vi "Demo HAL Tester LITE Auto.vi"() -> ()   [LabVIEW 2014]
doc: "Use this template to build a producer/consumer design pattern with events to produce queue items. Use this design pattern instead of the User Interface Event Handler pattern for user interfaces when you want to execute code asynchronously in response to an event without slowing the user interface responsiveness."
uses:
  TypeDefs/HAL Config Data.ctl
  APIs/Message Queue/Enqueue Message (Single).vi
  APIs/Message Queue/Enqueue Message (Array).vi
  APIs/Message Queue/WINFAS 2 Message Queue.lvlib
  HWSyncLoop/HWSyncLoop.lvlib
  APIs/Data Queue/WINFAS 2 Data Queue.lvlib
  HWAsyncLoop/HWAsyncLoop.lvlib
panel:
  out "Asyncs":string[][](array[string])
  out "Syncs":string[](array[string])
  out "Async Data":sgl[](array[numeric])
  in  "HWAsync CMD":bool
  in  "HWSync CMD":bool
  in  "Stop Cycle":bool
  in  "Start Cycle":bool
  in  "Config":bool
  in  "LOAD DRIVER":bool
  in  "Disconnect":bool
  in  "Connect":bool
  out "UI Mssge Log":string
  out "TDX":sgl[][](graph)
  out "Encoder":sgl[](array[slide]) scale=-3600.0..3600.0
  out "DO":bool[][](array[boolean])
  out "DI":bool[][](array[boolean])
  out "TDX ALL":string[][](table)
  out "HWSyncLog 1":string
  out "HWSyncLog 2":string
  out "HWSyncLog 3":string
  out "HWSyncLog 4":string
  out "HWSyncLog 5":string
  out "HWAsyncLogAll":string
  # "Entradas Digitales (0-15)"
  # "Salidas Digitales (0-15)"
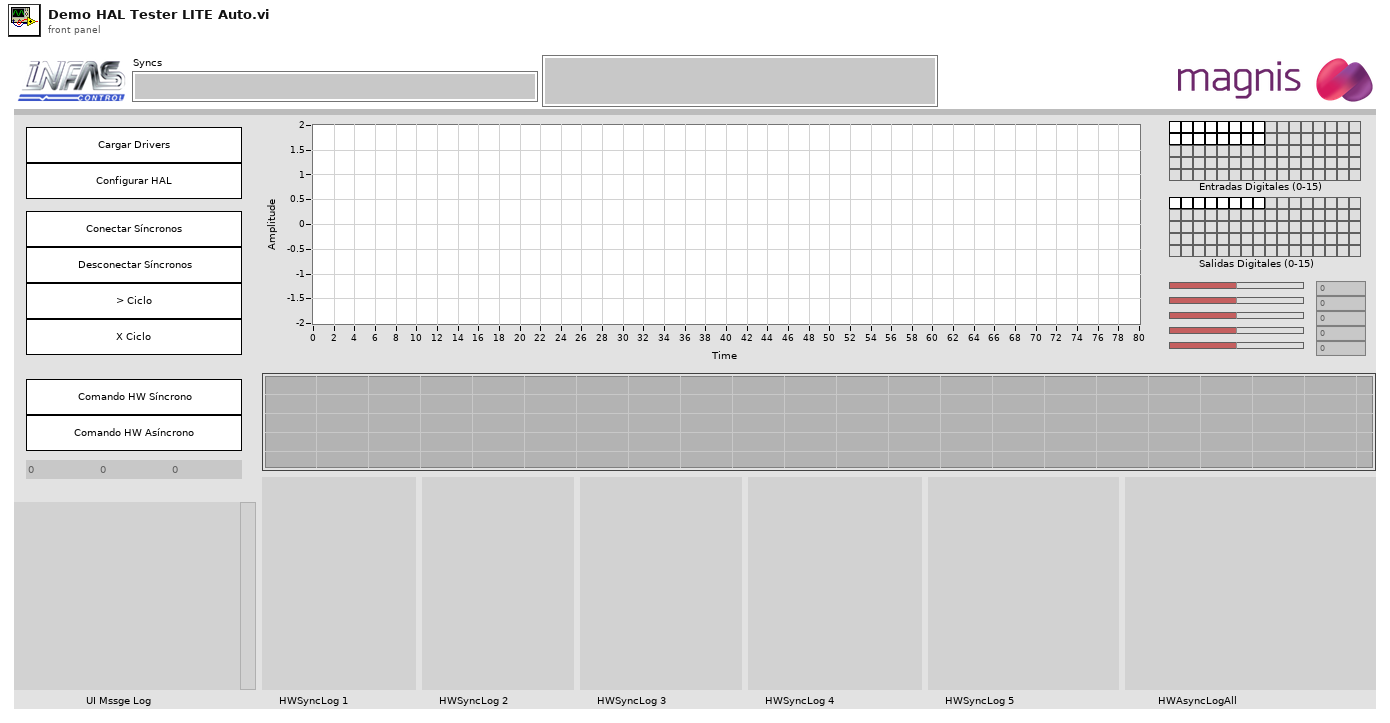
[diagram p1: front panel]
types:
  T1 = typedef "HAL Config Data.ctl" = cluster{"HWSync Index":u32, "Driver Name":string, "Channel Mask":u64}
  T2 = enum32{"invalid app kind", "Development System", "Run Time System", "Student Edition", "Embedded LabVIEW", "Evaluation", "Custom"}
  T3 = typedef "WINFAS 2 Message Queue.lvlib/All Message Queues.ctl" = cluster{"CORE":refnum<queue>, "Event UI":refnum<queue>, "Display UI":refnum<queue>, "MATH":refnum<queue>, "SEQ":refnum<queue>, "DB":refnum<queue>, "ERR":refnum<queue>, "HAL":refnum<queue>, "HWSync1":refnum<queue>, "HWSync2":refnum<queue>, "HWSync3":refnum<queue>, "HWSync4":refnum<queue>, "HWSync5":refnum<queue>, "HWAsync1":refnum<queue>, "HWAsync2":refnum<queue>, "HWAsync3":refnum<queue>, "HWAsync4":refnum<queue>, "HWAsync5":refnum<queue>, "HWAsync6":refnum<queue>, "HWAsync7":refnum<queue>, "HWAsync8":refnum<queue>, "HWAsync9":refnum<queue>, "HWAsync10":refnum<queue>}
  T4 = typedef "WINFAS 2 Data Queue.lvlib/All Data Queues Cluster.ctl" = cluster{"Queues":cluster{"ACQ HWSync1":refnum<queue>, "ACQ HWSync2":refnum<queue>, "ACQ HWSync3":refnum<queue>, "ACQ HWSync4":refnum<queue>, "ACQ HWSync5":refnum<queue>}, "Notifiers":cluster{"Control":cluster{"CTRL HWSync1":refnum<notifier>, "CTRL HWSync2":refnum<notifier>, "CTRL HWSync3":refnum<notifier>, "CTRL HWSync4":refnum<notifier>, "CTRL HWSync5":refnum<notifier>}, "Acquisition":cluster{"ACQ HWSync1":refnum<notifier>, "ACQ HWSync2":refnum<notifier>, "ACQ HWSync3":refnum<notifier>, "ACQ HWSync4":refnum<notifier>, "ACQ HWSync5":refnum<notifier>}, "Async":cluster{"ACQ HWAsync1":refnum<notifier>, "ACQ HWAsync2":refnum<notifier>, "ACQ HWAsync3":refnum<notifier>, "ACQ HWAsync4":refnum<notifier>, "ACQ HWAsync5":refnum<notifier>, "ACQ HWAsync6":refnum<notifier>, "ACQ HWAsync7":refnum<notifier>, "ACQ HWAsync8":refnum<notifier>, "ACQ HWAsync9":refnum<notifier>, "ACQ HWAsync10":refnum<notifier>}}}
  T5 = cluster{"ACQ HWSync1":refnum<notifier>, "ACQ HWSync2":refnum<notifier>, "ACQ HWSync3":refnum<notifier>, "ACQ HWSync4":refnum<notifier>, "ACQ HWSync5":refnum<notifier>}
  T6 = cluster{"CTRL HWSync1":refnum<notifier>, "CTRL HWSync2":refnum<notifier>, "CTRL HWSync3":refnum<notifier>, "CTRL HWSync4":refnum<notifier>, "CTRL HWSync5":refnum<notifier>}
  T7 = cluster{"ACQ HWSync1":refnum<queue>, "ACQ HWSync2":refnum<queue>, "ACQ HWSync3":refnum<queue>, "ACQ HWSync4":refnum<queue>, "ACQ HWSync5":refnum<queue>}
  T8 = cluster{"HWSync1":refnum<queue>, "HWSync2":refnum<queue>, "HWSync3":refnum<queue>, "HWSync4":refnum<queue>, "HWSync5":refnum<queue>}
  T9 = cluster{"HWAsync1":refnum<queue>, "HWAsync2":refnum<queue>, "HWAsync3":refnum<queue>, "HWAsync4":refnum<queue>, "HWAsync5":refnum<queue>, "HWAsync6":refnum<queue>, "HWAsync7":refnum<queue>, "HWAsync8":refnum<queue>, "HWAsync9":refnum<queue>, "HWAsync10":refnum<queue>}
  T10 = typedef "WINFAS 2 Data Queue.lvlib/Async Acquisition Data Cluster.ctl" = cluster{"Data":sgl[]}
  T11 = typedef "WINFAS 2 Data Queue.lvlib/Acquisition Data 1 Sample Cluster.ctl" = cluster{"TDX":sgl[], "Encoder":sgl}
  T12 = typedef "WINFAS 2 Data Queue.lvlib/Control Data Cluster.ctl" = cluster{"Encoder":sgl, "DI":bool[], "DO":bool[]}
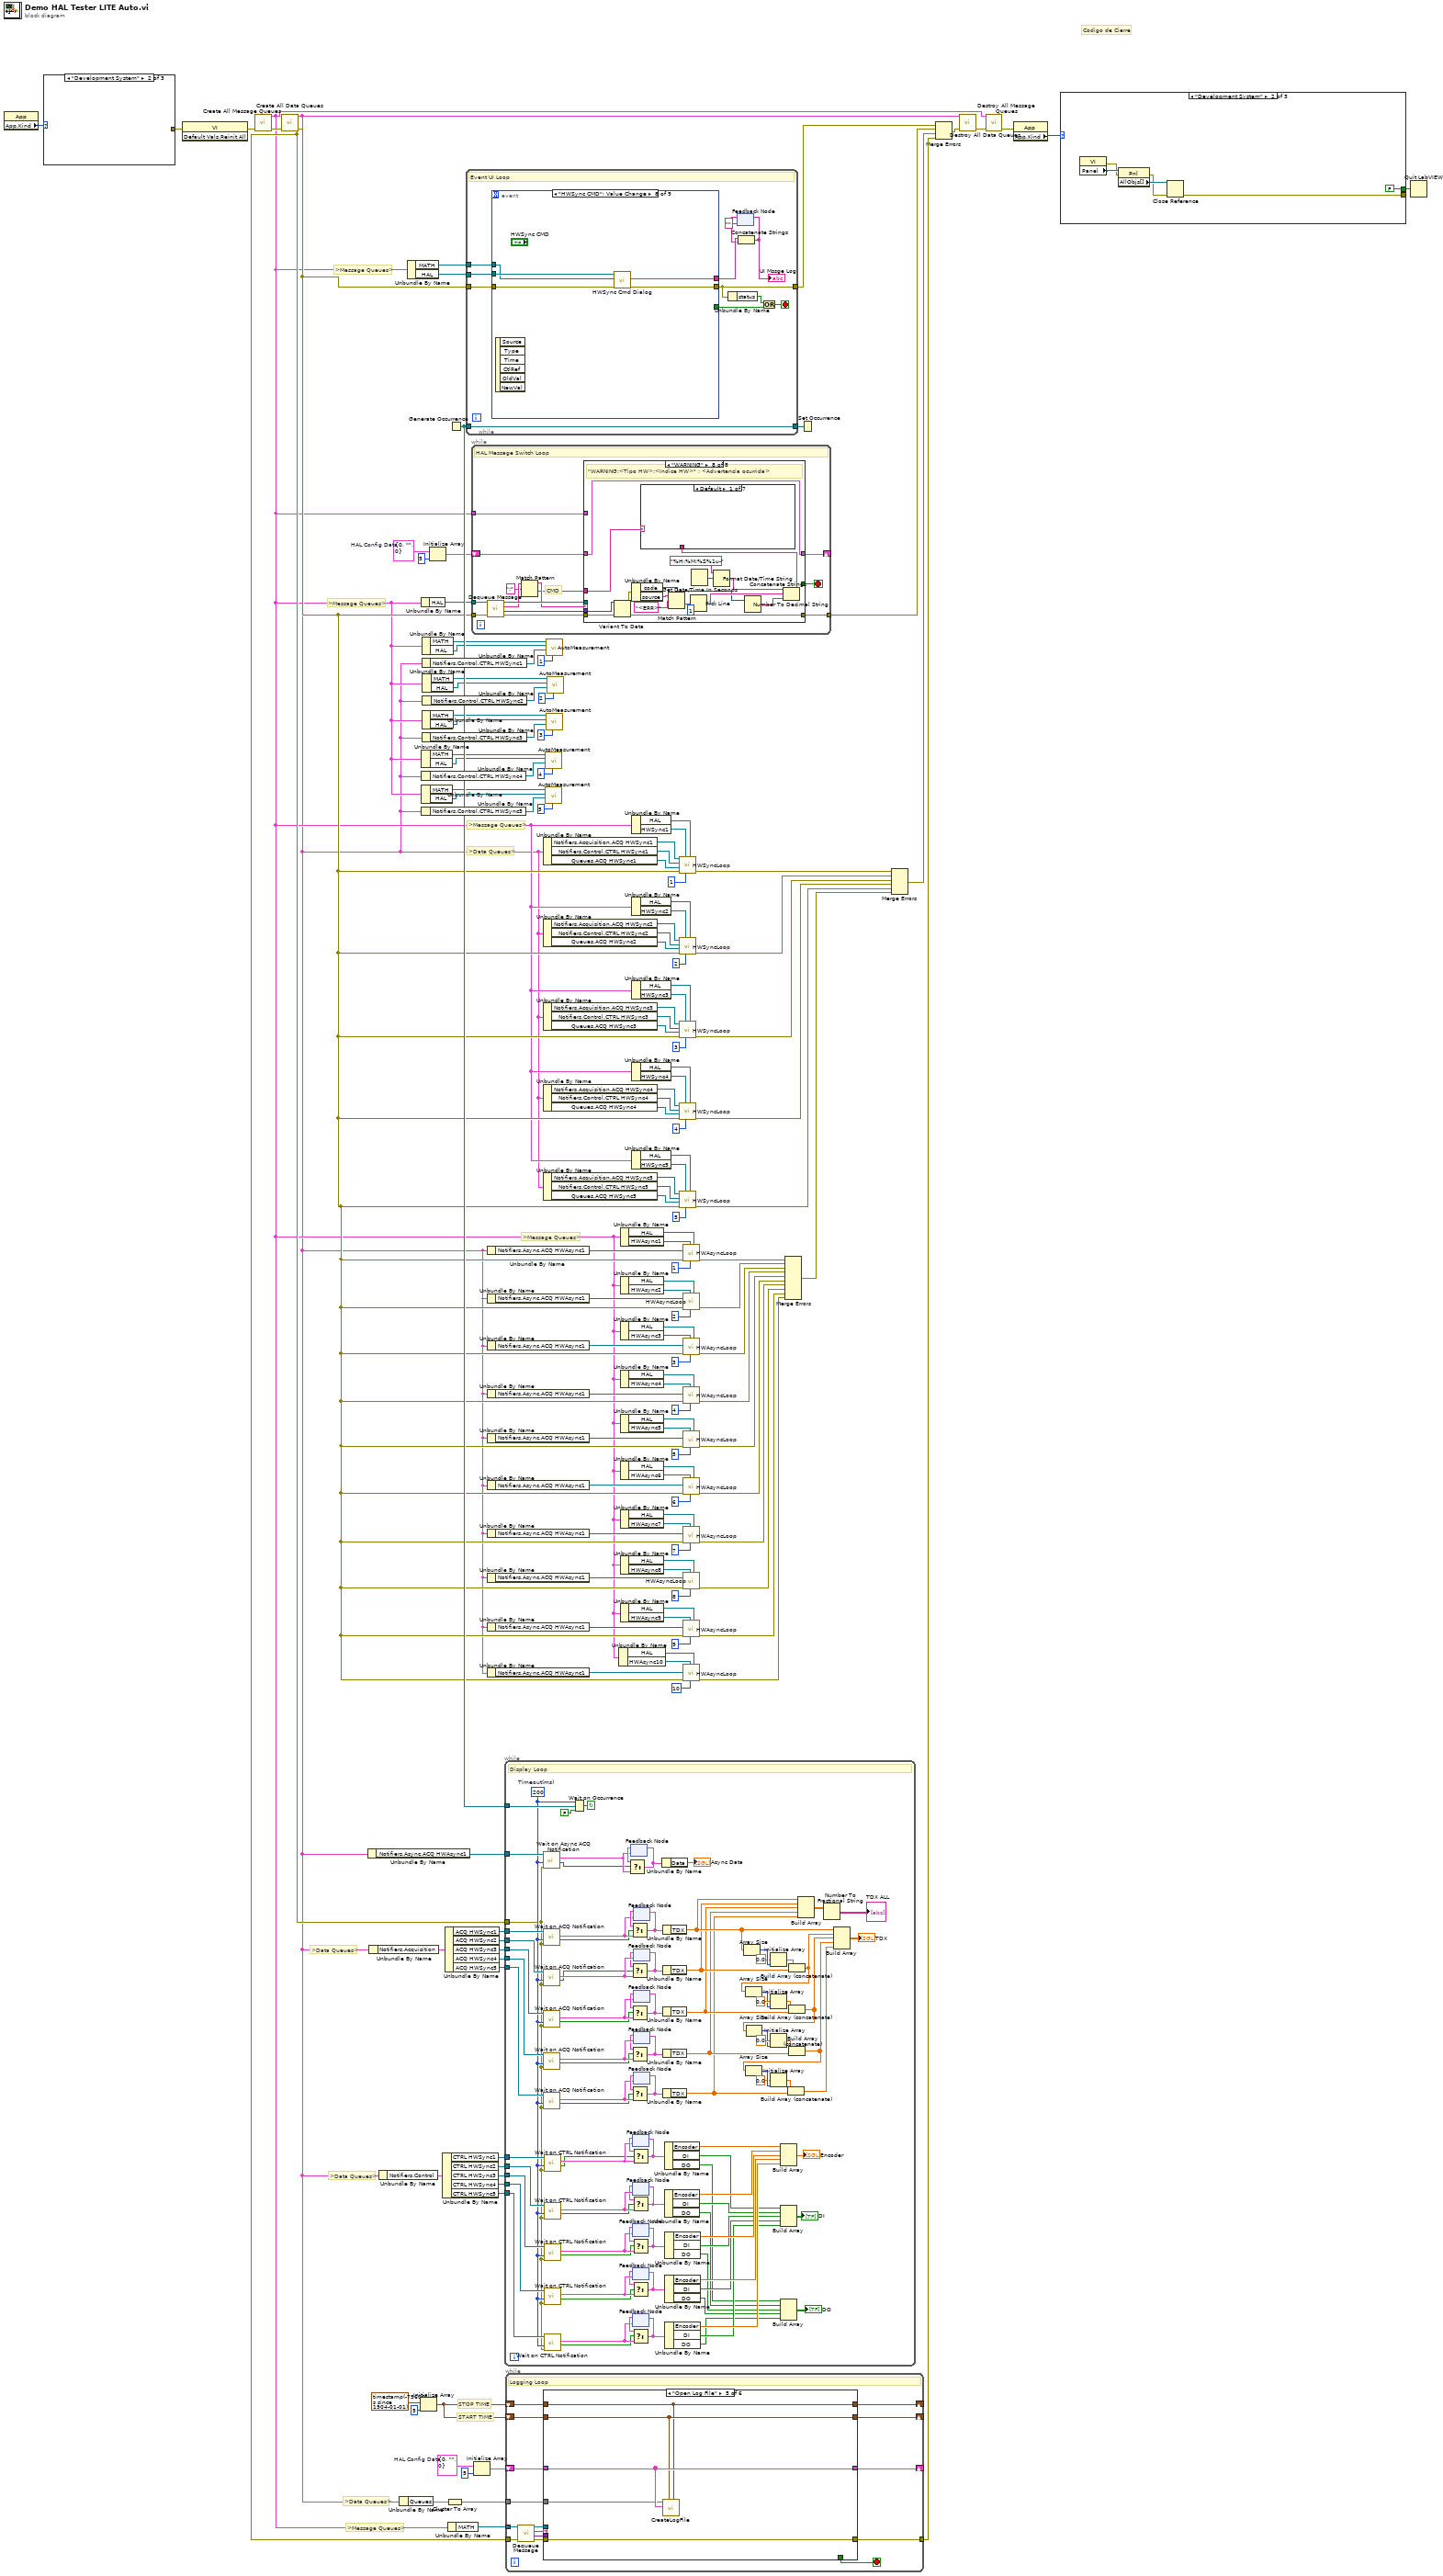
[diagram p0: block diagram]
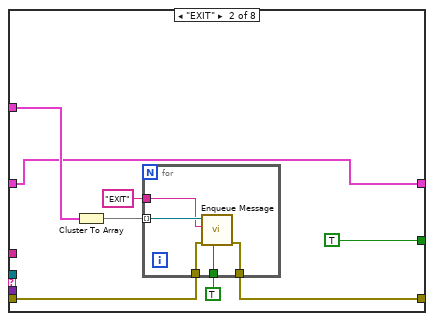
[diagram p3: hidden frame]
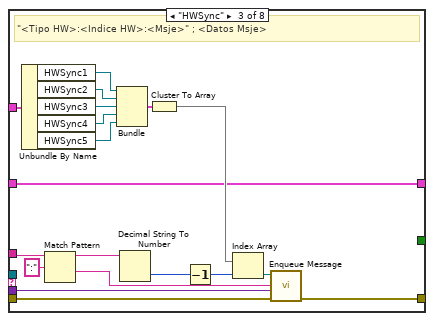
[diagram p4: hidden frame]
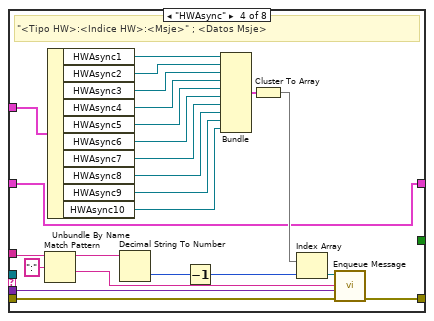
[diagram p5: hidden frame]
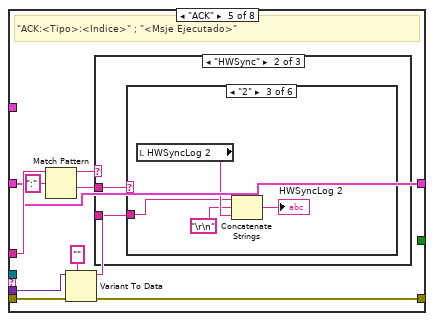
[diagram p6: hidden frame]
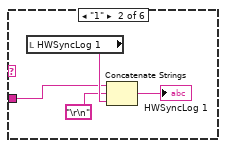
[diagram p9: hidden frame]
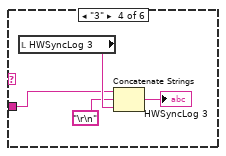
[diagram p10: hidden frame]
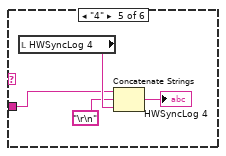
[diagram p11: hidden frame]
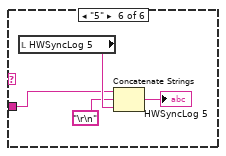
[diagram p12: hidden frame]
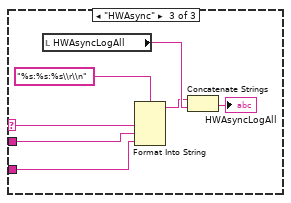
[diagram p13: hidden frame]
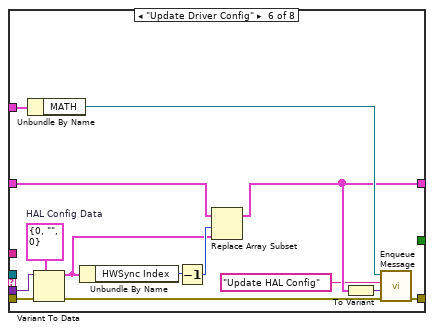
[diagram p14: hidden frame]
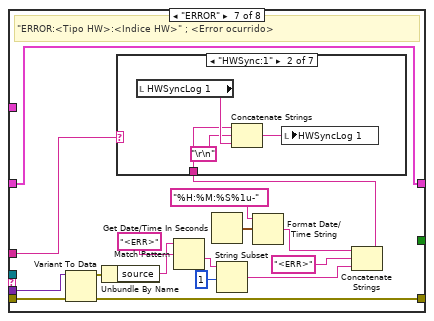
[diagram p15: hidden frame]
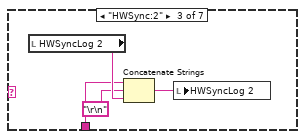
[diagram p17: hidden frame]
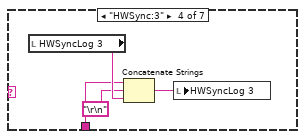
[diagram p18: hidden frame]
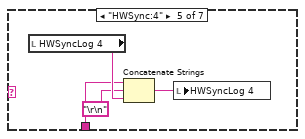
[diagram p19: hidden frame]
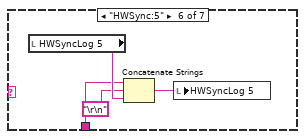
[diagram p20: hidden frame]
diagram:
  w39 = T1 {"HWSync Index"=0, "Driver Name"="", "Channel Mask"=0}  # HAL Config Data
  w42 = T1 {"HWSync Index"=0, "Driver Name"="", "Channel Mask"=0}  # HAL Config Data
  # "START TIME"
  # "STOP TIME"
  # ">Message Queues>"
  # ">Message Queues>"
  # ">Data Queues>"
  # "Codigo de Cierre"
  # ">Message Queues>"
  # ">Data Queues>"
  # ">Message Queues>"
  # ">Data Queues>"
  # ">Data Queues>"
  # ">Message Queues>"
  n1 = property class="App"() -> ("App.Kind"=w143:T2)  [unwired: 2 in, 2 out]
  n2 = case shown="\"Development System\"" w143 {
    tunnel: [_ _ w154] -> w142
    frame "invalid app kind", Default {
    }
    frame "Development System" {
    }
    frame "Run Time System" {
      w153 = FALSE ("Front Panel Window:Show Menu Bar")
      n3 = invoke class="VI" method="FP.Run-Time Position.Maximized"("Monitor"=i16 0) -> (error out=w154:errorcluster)  [unwired: 3 in, 3 out]
      n4 = property class="VI"("Front Panel.ShowMenuBar"=w153, "TB.Visible"=w153) -> ()  [unwired: 2 in, 2 out]
    }
  }
  n5 = invoke class="VI" method="Default Vals.Reinit All"(error in=w142) -> (error out=w133:errorcluster)  [unwired: 2 in, 2 out]
  n6 = call "Create All Message Queues.vi"("error in (no error)"=w133) -> ("error out"=w134:errorcluster, "Message Queues Out"=w2:T3)  [unwired: 9 in]
  n7 = call "Create All Data Queues.vi"("Error In"=w134) -> ("Error Out"=w57:errorcluster, "WINFAS 2 Data Queue.lvlib:All Data Queues Cluster"=w1:T4)  [unwired: 9 in]
  n8 = Unbundle By Name(w1) -> ("Notifiers.Async.ACQ HWAsync1"=w24:refnum<notifier>)
  n9 = Unbundle By Name(w1) -> ("Notifiers.Acquisition"=w89:T5)
  n10 = Unbundle By Name(w1) -> ("Notifiers.Control"=w88:T6)
  n11 = Unbundle By Name(w1) -> ("Queues"=w36:T7)
  n12 = Unbundle By Name(w2) -> ("MATH"=w152:refnum<queue>, "HAL"=w148:refnum<queue>)
  n13 = Initialize Array(timestamp(-75600 s since 1904-01-01) ("current time"), 5 ("dimension size")) -> (w43:timestamp[])
  n14 = Unbundle By Name(w2) -> ("HAL"=w23:refnum<queue>)
  n15 = Unbundle By Name(w2) -> ("MATH"=w7:refnum<queue>, "HAL"=w8:refnum<queue>)
  n16 = Unbundle By Name(w1) -> ("Notifiers.Control.CTRL HWSync4"=w9:refnum<notifier>)
  n17 = Unbundle By Name(w2) -> ("MATH"=w6:refnum<queue>, "HAL"=w5:refnum<queue>)
  n18 = Unbundle By Name(w1) -> ("Notifiers.Control.CTRL HWSync5"=w4:refnum<notifier>)
  n19 = Unbundle By Name(w2) -> ("MATH"=w22:refnum<queue>, "HAL"=w21:refnum<queue>)
  n20 = Unbundle By Name(w1) -> ("Notifiers.Control.CTRL HWSync1"=w20:refnum<notifier>)
  n21 = Unbundle By Name(w2) -> ("MATH"=w14:refnum<queue>, "HAL"=w13:refnum<queue>)
  n22 = Unbundle By Name(w1) -> ("Notifiers.Control.CTRL HWSync3"=w12:refnum<notifier>)
  n23 = Unbundle By Name(w2) -> ("MATH"=w15:refnum<queue>, "HAL"=w16:refnum<queue>)
  n24 = Unbundle By Name(w1) -> ("Notifiers.Control.CTRL HWSync2"=w17:refnum<notifier>)
  n25 = Initialize Array(w39, 5 ("dimension size")) -> (w37:T1[])
  n26 = Unbundle By Name(w88) -> ("CTRL HWSync1"=w97:refnum<notifier>, "CTRL HWSync2"=w96:refnum<notifier>, "CTRL HWSync3"=w95:refnum<notifier>, "CTRL HWSync4"=w94:refnum<notifier>, "CTRL HWSync5"=w93:refnum<notifier>)
  n27 = Unbundle By Name(w89) -> ("ACQ HWSync1"=w138:refnum<notifier>, "ACQ HWSync2"=w101:refnum<notifier>, "ACQ HWSync3"=w100:refnum<notifier>, "ACQ HWSync4"=w99:refnum<notifier>, "ACQ HWSync5"=w98:refnum<notifier>)
  n28 = Cluster To Array(cluster=w36) -> (array=w35:refnum<queue>[])
  n29 = Unbundle By Name(w2) -> ("MATH"=w146:refnum<queue>)
  n30 = Generate Occurrence() -> (w131:refnum<k4>)
  n31 = while {
    tunnel: w152 -> [w167]
    tunnel: w148 -> [w162]
    tunnel: [w160] -> w132
    tunnel: w131 -> [w160]
    tunnel: w57 -> [w166]
    tunnel: [w164] -> w149
    stop <- w161 stop-if-true
    # "Event UI Loop"
    n32 = event shown="[7] \"HWSync CMD\": Value Change" {
      selector: _ -> [_ _ _ _ _ _ _ _ _]
      dyn-events: _ -> [_ _ _ _ _ _ _ _ _]
      timeout: _ -> [_ _ _ _ _ _ _ _ _]
      tunnel: w167 -> [w173 _ _ _ _ _ w232 w247 _]
      tunnel: w166 -> [w175 w185 w191 w200 w207 w214 w231 w251 w257]
      tunnel: [w170 w183 w190 w199 w206 w212 w236 w250 w255] -> w164
      tunnel: [TRUE ("stop") _ _ _ _ _ _ _ _] -> w165
      tunnel: w162 -> [w176 w184 w189 w198 w205 w213 w237 w249 w252]
      tunnel: [_ w182 w186 w195 w204 w209 w235 w248 w254] -> w159
      event Panel Close? {
        w174 = TRUE ("Priority Message? (F)")
        w172 = "EXIT" ("String")
        n33 = event-data() -> ()  [unwired: 1 in, 1 out]
        n34 = call-poly "Enqueue Message.vi"("Priority Message? (F)"=w174, "error in (no error)"=w175, "Message"=w172, "Message Queue"=w176) -> ("error out"=w171:errorcluster)  [unwired: 6 in, 1 out]
        n35 = call-poly "Enqueue Message.vi"("Priority Message? (F)"=w174, "error in (no error)"=w171, "Message"=w172, "Message Queue"=w173) -> ("error out"=w170:errorcluster)  [unwired: 6 in, 1 out]
        n36 = event-data("Discard?"=TRUE) -> ()  [unwired: 1 in, 1 out]
      }
      event "LOAD DRIVER": Value Change {
        n37 = event-data() -> ()  [unwired: 1 in, 1 out]
        n38 = call "Load Drivers Dialog.vi"("error in (no error)"=w185, "Message Queue in"=w184) -> ("error out"=w183:errorcluster, "Mssgs Sent"=w182:string, "Asyncs"=w180:string[], "Syncs"=→"Syncs":string[])  [unwired: 6 in]
        n39 = Reshape Array(w180, 2 ("dimension size"), 5 ("dimension size")) -> (→"Asyncs":string[][])
      }
      event "Connect": Value Change {
        w188 = string[] ["HWSync:1:Port:Open", "HWSync:2:Port:Open", "HWSync:3:Port:Open", "HWSync:4:Port:Open", "HWSync:5:Port:Open"] ("Message Array")
        n40 = event-data() -> ()  [unwired: 1 in, 1 out]
        n41 = for {
          tunnel: [w194] -> w187 mode=indexing
          tunnel: w188 -> [w193] mode=indexing
          n42 = Concatenate Strings(w193, "\r\n") -> (w194:string)
        }
        n43 = call-poly "Enqueue Message.vi"("error in (no error)"=w191, "Message Array"=w188, "Message Queue"=w189) -> ("error out"=w190:errorcluster)  [unwired: 7 in, 1 out]
        n44 = Concatenate Strings(w187) -> (w186:string)
      }
      event "Disconnect": Value Change {
        w196 = string[] ["HWSync:1:Port:Close", "HWSync:2:Port:Close", "HWSync:3:Port:Close", "HWSync:4:Port:Close", "HWSync:5:Port:Close"] ("Message Array")
        n45 = event-data() -> ()  [unwired: 1 in, 1 out]
        n46 = for {
          tunnel: [w203] -> w197 mode=indexing
          tunnel: w196 -> [w202] mode=indexing
          n47 = Concatenate Strings(w202, "\r\n") -> (w203:string)
        }
        n48 = call-poly "Enqueue Message.vi"("error in (no error)"=w200, "Message Array"=w196, "Message Queue"=w198) -> ("error out"=w199:errorcluster)  [unwired: 7 in, 1 out]
        n49 = Concatenate Strings(w197) -> (w195:string)
      }
      event "Config": Value Change {
        n50 = event-data() -> ()  [unwired: 1 in, 1 out]
        n51 = call "Config Select Dialog.vi"("Error In"=w207, "Message Queue"=w205) -> ("Error Out"=w206:errorcluster, "Msg out"=w204:string)  [unwired: 8 in]
      }
      event "Start Cycle": Value Change {
        n52 = event-data() -> ()  [unwired: 1 in, 2 out]
        n53 = for {
          N: 5 -> [_]
          tunnel: w213 -> [w228]
          shift-right: [w227] -> w212
          shift-left: w214 -> [w229]
          tunnel: [w218] -> w210 mode=concatenating
          i -> [w226]
          n54 = Increment(x=w226) -> (x+1=w222:i32)
          n55 = Format Into String(format string="HWSync:%d:Auto-Refresh:Init" ("String"), w222) -> (resulting string=w221:string)  [unwired: 2 in, 1 out]
          n56 = Format Into String(format string="HWSync:%d:Auto-Refresh:Start" ("String"), w222) -> (resulting string=w220:string)  [unwired: 2 in, 1 out]
          n57 = Format Into String(format string="HWSync:%d:Diagnostic:Cycle" ("String"), w222) -> (resulting string=w219:string)  [unwired: 2 in, 1 out]
          n58 = Build Array(w221, w220, w219) -> (w218:string[])
          n59 = call-poly "Enqueue Message.vi"("error in (no error)"=w229, "Message Array"=w218, "Message Queue"=w228) -> ("error out"=w227:errorcluster)  [unwired: 7 in, 1 out]
        }
        n60 = for {
          tunnel: [w217] -> w211 mode=indexing
          tunnel: w210 -> [w216] mode=indexing
          n61 = Concatenate Strings(w216, "\r\n") -> (w217:string)
        }
        n62 = Concatenate Strings(w211) -> (w209:string)
      }
      event "Stop Cycle": Value Change {
        n63 = event-data() -> ()  [unwired: 1 in, 1 out]
        n64 = for {
          N: 5 -> [_]
          tunnel: w237 -> [w245]
          shift-right: [w244] -> w236
          shift-left: w231 -> [w246]
          tunnel: [w238] -> w234 mode=indexing
          i -> [w243]
          n65 = Increment(x=w243) -> (x+1=w241:i32)
          n66 = Format Into String(format string="HWSync:%d:Auto-Refresh:Stop" ("String"), w241) -> (resulting string=w239:string)  [unwired: 2 in, 1 out]
          n67 = call-poly "Enqueue Message.vi"("error in (no error)"=w246, "Message"=w239, "Message Queue"=w245) -> ("error out"=w244:errorcluster)  [unwired: 7 in, 1 out]
          n68 = Concatenate Strings(w239, "\r\n") -> (w238:string)
        }
        n69 = call-poly "Enqueue Message.vi"("error in (no error)"=w231, "Message"="Open Log File", "Message Queue"=w232) -> ()  [unwired: 7 in, 2 out]
        n70 = Concatenate Strings(w234) -> (w235:string)
      }
      event "HWSync CMD": Value Change {
        n71 = event-data() -> ()  [unwired: 1 in, 6 out]
        n72 = call "HWSync Cmd Dialog.vi"("error in (no error)"=w251, "Log Queue"=w247, "Hal Queue in"=w249) -> ("error out"=w250:errorcluster, "Msg out"=w248:string)  [unwired: 7 in]
      }
      event "HWAsync CMD": Value Change {
        n73 = event-data() -> ()  [unwired: 1 in, 6 out]
        n74 = call "HWAsync Cmd Dialog.vi"("error in (no error)"=w257) -> ("error out"=w256:errorcluster, "Msg out"=w253:string)  [unwired: 9 in]
        n75 = call "HWAsync Cmd END Dialog.vi"("error in (no error)"=w256, "Msg in"=w253, "Message Queue"=w252) -> ("error out"=w255:errorcluster, "Msg out"=w254:string)  [unwired: 7 in]
      }
    }
    n76 = Unbundle By Name(w164) -> ("status"=w163:bool)
    n77 = feedback #1("") -> (w158:string)
    n78 = Concatenate Strings(w159, w158) -> (w157:string)
    "UI Mssge Log" <- w157
    n79 = feedback-in #1(w157) -> ()
    n80 = Or(x=w163, y=w165) -> (x .or. y?=w161:bool)
  }
  n81 = while {
    tunnel: w23 -> [w271]
    tunnel: w57 -> [w270]
    tunnel: [w262] -> w90
    tunnel: w2 -> [w261]
    shift-right: [w258] -> _
    shift-left: w37 -> [w259]
    stop <- w266 stop-if-true
    # "CMD"
    # "HAL Message Switch Loop"
    n82 = call "Dequeue Message.vi"("error in (no error)"=w270, "Message Queue"=w271) -> ("error out"=w269:errorcluster, "Message Data"=w268:variant, "Message"=w265:string, "dup Message Queue"=w267:refnum<queue>)  [unwired: 6 in]
    n83 = Match Pattern(string=w265, regular expression=":") -> (before substring=w263:string, after substring=w260:string)  [unwired: 1 in, 2 out]
    n84 = case shown="\"WARNING\"" w263 {
      tunnel: w269 -> [w273 w280 w305 w329 w339 w382 w389 w436]
      tunnel: w268 -> [_ _ w303 w327 w338 w381 w398 w441]
      tunnel: w267 -> [_ _ _ _ _ _ _ _]
      tunnel: [_ TRUE _ _ _ _ _ _] -> w266
      tunnel: [w273 w279 w304 w328 w337 w374 w397 w440] -> w262
      tunnel: w261 -> [_ w277 w302 w326 _ w373 _ _]
      tunnel: w260 -> [_ _ w295 w320 w333 _ w386 w434]
      tunnel: w259 -> [w272 w274 w287 w306 w330 w376 w385 w433]
      tunnel: [w272 w274 w287 w306 w330 w370 w385 w433] -> w258
      frame Default {
      }
      frame "EXIT" {
        n85 = Cluster To Array(cluster=w277) -> (array=w276:refnum<queue>[])
        n86 = for {
          tunnel: w276 -> [w284] mode=indexing
          tunnel: "EXIT" ("regular expression") -> [w283]
          tunnel: w280 -> [w286]
          tunnel: [w285] -> w279
          tunnel: TRUE -> [w282]
          n87 = call-poly "Enqueue Message.vi"("Priority Message? (F)"=w282, "error in (no error)"=w286, "Message"=w283, "Message Queue"=w284) -> ("error out"=w285:errorcluster)  [unwired: 6 in, 1 out]
        }
      }
      frame "HWSync" {
        # "\"<Tipo HW>:<Indice HW>:<Msje>\" ; <Datos Msje>"
        n88 = Unbundle By Name(w302) -> ("HWSync1"=w298:refnum<queue>, "HWSync2"=w300:refnum<queue>, "HWSync3"=w301:refnum<queue>, "HWSync4"=w299:refnum<queue>, "HWSync5"=w297:refnum<queue>)
        n89 = Match Pattern(string=w295, regular expression=":") -> (before substring=w292:string, after substring=w290:string)  [unwired: 1 in, 2 out]
        n90 = Bundle("HWSync1"=w298, "HWSync2"=w300, "HWSync3"=w301, "HWSync4"=w299, "HWSync5"=w297) -> (w294:T8)  [unwired: 1 in]
        n91 = Decimal String To Number(string=w292) -> (number=w288:i32)  [unwired: 2 in, 1 out]
        n92 = Cluster To Array(cluster=w294) -> (array=w293:refnum<queue>[])
        n93 = Decrement(x=w288) -> (x-1=w289:i32)
        n94 = Index Array(array=w293, index=w289) -> (element=w291:refnum<queue>)
        n95 = call-poly "Enqueue Message.vi"("error in (no error)"=w305, "Message Data"=w303, "Message"=w290, "Message Queue"=w291) -> ("error out"=w304:errorcluster)  [unwired: 6 in, 1 out]
      }
      frame "HWAsync" {
        # "\"<Tipo HW>:<Indice HW>:<Msje>\" ; <Datos Msje>"
        n96 = Match Pattern(string=w320, regular expression=":") -> (before substring=w317:string, after substring=w315:string)  [unwired: 1 in, 2 out]
        n97 = Unbundle By Name(w326) -> ("HWAsync1"=w323:refnum<queue>, "HWAsync2"=w307:refnum<queue>, "HWAsync3"=w325:refnum<queue>, "HWAsync4"=w324:refnum<queue>, "HWAsync5"=w322:refnum<queue>, "HWAsync6"=w308:refnum<queue>, "HWAsync7"=w309:refnum<queue>, "HWAsync8"=w310:refnum<queue>, "HWAsync9"=w311:refnum<queue>, "HWAsync10"=w312:refnum<queue>)
        n98 = Decimal String To Number(string=w317) -> (number=w313:i32)  [unwired: 2 in, 1 out]
        n99 = Decrement(x=w313) -> (x-1=w314:i32)
        n100 = Bundle("HWAsync1"=w323, "HWAsync2"=w307, "HWAsync3"=w325, "HWAsync4"=w324, "HWAsync5"=w322, "HWAsync6"=w308, "HWAsync7"=w309, "HWAsync8"=w310, "HWAsync9"=w311, "HWAsync10"=w312) -> (w319:T9)  [unwired: 1 in]
        n101 = Cluster To Array(cluster=w319) -> (array=w318:refnum<queue>[])
        n102 = Index Array(array=w318, index=w314) -> (element=w316:refnum<queue>)
        n103 = call-poly "Enqueue Message.vi"("error in (no error)"=w329, "Message Data"=w327, "Message"=w315, "Message Queue"=w316) -> ("error out"=w328:errorcluster)  [unwired: 6 in, 1 out]
      }
      frame "ACK" {
        # "\"ACK:<Tipo>:<Indice>\" ; \"<Msje Ejecutado>\""
        n104 = Match Pattern(string=w333, regular expression=":") -> (before substring=w334:string, after substring=w331:string)  [unwired: 1 in, 2 out]
        n105 = Variant To Data(error in=w339, type="", Variant=w338) -> (data=w336:string, error out=w337:errorcluster)
        n106 = case shown="\"HWSync\"" w334 {
          selector: w334 -> [_ _ w367]
          tunnel: w336 -> [_ w341 w365]
          tunnel: w331 -> [_ w340 w366]
          frame Default {
          }
          frame "HWSync" {
            n107 = case shown="\"2\"" w340 {
              tunnel: w341 -> [_ w342 w348 w352 w356 w360]
              frame Default {
              }
              frame "1" {
                n108 = local read "HWSyncLog 1"() -> (w345:string)
                n109 = Concatenate Strings(w342, "\r\n", w345) -> (→"HWSyncLog 1":string)
              }
              frame "2" {
                n110 = local read "HWSyncLog 2"() -> (w349:string)
                n111 = Concatenate Strings(w348, "\r\n", w349) -> (→"HWSyncLog 2":string)
              }
              frame "3" {
                n112 = local read "HWSyncLog 3"() -> (w353:string)
                n113 = Concatenate Strings(w352, "\r\n", w353) -> (→"HWSyncLog 3":string)
              }
              frame "4" {
                n114 = local read "HWSyncLog 4"() -> (w357:string)
                n115 = Concatenate Strings(w356, "\r\n", w357) -> (→"HWSyncLog 4":string)
              }
              frame "5" {
                n116 = local read "HWSyncLog 5"() -> (w361:string)
                n117 = Concatenate Strings(w360, "\r\n", w361) -> (→"HWSyncLog 5":string)
              }
            }
          }
          frame "HWAsync" {
            n118 = local read "HWAsyncLogAll"() -> (w364:string)
            n119 = Format Into String(format string="%s:%s:%s\\r\\n", w367, w366, w365) -> (resulting string=w363:string)  [unwired: 2 in, 1 out]
            n120 = Concatenate Strings(w363, w364) -> (→"HWAsyncLogAll":string)
          }
        }
      }
      frame "Update Driver Config" {
        w380 = T1 {"HWSync Index"=0, "Driver Name"="", "Channel Mask"=0}  # HAL Config Data
        n121 = Unbundle By Name(w373) -> ("MATH"=w372:refnum<queue>)
        n122 = Variant To Data(error in=w382, type=w380, Variant=w381) -> (data=w377:T1, error out=w375:errorcluster)
        n123 = Unbundle By Name(w377) -> ("HWSync Index"=w379:u32)
        n124 = Decrement(x=w379) -> (x-1=w378:u32)
        n125 = Replace Array Subset(array=w376, new element=w377, index=w378) -> (w370:T1[])
        n126 = To Variant(anything=w370) -> (Variant=w371:variant)
        n127 = call-poly "Enqueue Message.vi"("error in (no error)"=w375, "Message Data"=w371, "Message"="Update HAL Config" ("regular expression"), "Message Queue"=w372) -> ("error out"=w374:errorcluster)  [unwired: 6 in, 1 out]
      }
      frame "ERROR" {
        # "\"ERROR:<Tipo HW>:<Indice HW>\" ; <Error ocurrido>"
        n128 = Variant To Data(error in=w389, type=w389, Variant=w398) -> (data=w388:errorcluster, error out=w397:errorcluster)
        n129 = Unbundle By Name(w388) -> ("source"=w395:string)
        n130 = Match Pattern(string=w395, regular expression="<ERR>") -> (after substring=w391:string)  [unwired: 1 in, 3 out]
        n131 = Get Date/Time In Seconds() -> (seconds since 1Jan1904=w394:timestamp)
        n132 = String Subset(string=w391, offset (0)=1) -> (substring=w384:string)  [unwired: 1 in]
        n133 = Format Date/Time String(time format string (%c)="%H:%M:%S%1u-", seconds (now)=w394) -> (date/time string=w392:string)  [unwired: 1 in]
        n134 = Concatenate Strings(w392, "<ERR>" ("string"), w384) -> (w387:string)
        n135 = case shown="\"HWSync:1\"" w386 {
          selector: w386 -> [_ _ _ _ _ _ w422]
          tunnel: w387 -> [_ w401 w405 w409 w413 w417 w424]
          frame Default {
          }
          frame "HWSync:1" {
            n136 = local read "HWSyncLog 1"() -> (w402:string)
            n137 = Concatenate Strings(w401, "\r\n", w402) -> (w399:string)
            n138 = local write "HWSyncLog 1"(w399) -> ()
          }
          frame "HWSync:2" {
            n139 = local read "HWSyncLog 2"() -> (w406:string)
            n140 = Concatenate Strings(w405, "\r\n", w406) -> (w403:string)
            n141 = local write "HWSyncLog 2"(w403) -> ()
          }
          frame "HWSync:3" {
            n142 = local read "HWSyncLog 3"() -> (w410:string)
            n143 = Concatenate Strings(w409, "\r\n", w410) -> (w407:string)
            n144 = local write "HWSyncLog 3"(w407) -> ()
          }
          frame "HWSync:4" {
            n145 = local read "HWSyncLog 4"() -> (w414:string)
            n146 = Concatenate Strings(w413, "\r\n", w414) -> (w411:string)
            n147 = local write "HWSyncLog 4"(w411) -> ()
          }
          frame "HWSync:5" {
            n148 = local read "HWSyncLog 5"() -> (w418:string)
            n149 = Concatenate Strings(w417, "\r\n", w418) -> (w415:string)
            n150 = local write "HWSyncLog 5"(w415) -> ()
          }
          frame "HWAsync:1", "HWAsync:10", "HWAsync:2", "HWAsync:3", "HWAsync:4", "HWAsync:5", "HWAsync:6", "HWAsync:7", "HWAsync:8", "HWAsync:9" {
            n151 = local read "HWAsyncLogAll"() -> (w419:string)
            n152 = Concatenate Strings(w422, ":" ("string"), w424, "\r\n", w419) -> (w420:string)
            n153 = local write "HWAsyncLogAll"(w420) -> ()
          }
        }
      }
      frame "WARNING" {
        # "\"WARNING:<Tipo HW>:<Indice HW>\" ; <Advertencia ocurrida>"
        n154 = Variant To Data(error in=w436, type=w436, Variant=w441) -> (data=w431:errorcluster, error out=w440:errorcluster)
        n155 = Unbundle By Name(w431) -> ("code"=w426:i32, "source"=w430:string)
        n156 = Match Pattern(string=w430, regular expression="<ERR>") -> (after substring=w428:string)  [unwired: 1 in, 3 out]
        n157 = Pick Line(multi-line string=w428, line index=1) -> (output string=w427:string)  [unwired: 1 in]
        n158 = Get Date/Time In Seconds() -> (seconds since 1Jan1904=w439:timestamp)
        n159 = Format Date/Time String(time format string (%c)="%H:%M:%S%1u-", seconds (now)=w439) -> (date/time string=w437:string)  [unwired: 1 in]
        n160 = Number To Decimal String(number=w426) -> (decimal integer string=w432:string)  [unwired: 1 in]
        n161 = Concatenate Strings(w437, w427, w432) -> (w435:string)
        n162 = case shown="Default" w434 {
          selector: w434 -> [_ _ _ _ _ _ w465]
          tunnel: w435 -> [_ w444 w448 w452 w456 w460 w467]
          frame Default {
          }
          frame "HWSync:1" {
            n163 = local read "HWSyncLog 1"() -> (w445:string)
            n164 = Concatenate Strings(w444, "\r\n", w445) -> (w442:string)
            n165 = local write "HWSyncLog 1"(w442) -> ()
          }
          frame "HWSync:2" {
            n166 = local read "HWSyncLog 2"() -> (w449:string)
            n167 = Concatenate Strings(w448, "\r\n", w449) -> (w446:string)
            n168 = local write "HWSyncLog 2"(w446) -> ()
          }
          frame "HWSync:3" {
            n169 = local read "HWSyncLog 3"() -> (w453:string)
            n170 = Concatenate Strings(w452, "\r\n", w453) -> (w450:string)
            n171 = local write "HWSyncLog 3"(w450) -> ()
          }
          frame "HWSync:4" {
            n172 = local read "HWSyncLog 4"() -> (w457:string)
            n173 = Concatenate Strings(w456, "\r\n", w457) -> (w454:string)
            n174 = local write "HWSyncLog 4"(w454) -> ()
          }
          frame "HWSync:5" {
            n175 = local read "HWSyncLog 5"() -> (w461:string)
            n176 = Concatenate Strings(w460, "\r\n", w461) -> (w458:string)
            n177 = local write "HWSyncLog 5"(w458) -> ()
          }
          frame "HWAsync:1", "HWAsync:10", "HWAsync:2", "HWAsync:3", "HWAsync:4", "HWAsync:5", "HWAsync:6", "HWAsync:7", "HWAsync:8", "HWAsync:9" {
            n178 = local read "HWAsyncLogAll"() -> (w462:string)
            n179 = Concatenate Strings(w465, ":" ("string"), w467, "\r\n", w462) -> (w463:string)
            n180 = local write "HWAsyncLogAll"(w463) -> ()
          }
        }
      }
    }
  }
  n181 = Initialize Array(w42, 5 ("dimension size")) -> (w40:T1[])
  n182 = Unbundle By Name(w1) -> ("Notifiers.Async.ACQ HWAsync1"=w34:refnum<notifier>)
  n183 = Unbundle By Name(w1) -> ("Notifiers.Async.ACQ HWAsync1"=w33:refnum<notifier>)
  n184 = Unbundle By Name(w1) -> ("Notifiers.Async.ACQ HWAsync1"=w32:refnum<notifier>)
  n185 = Unbundle By Name(w1) -> ("Notifiers.Async.ACQ HWAsync1"=w31:refnum<notifier>)
  n186 = Unbundle By Name(w1) -> ("Notifiers.Async.ACQ HWAsync1"=w30:refnum<notifier>)
  n187 = Unbundle By Name(w1) -> ("Notifiers.Async.ACQ HWAsync1"=w29:refnum<notifier>)
  n188 = Unbundle By Name(w1) -> ("Notifiers.Async.ACQ HWAsync1"=w28:refnum<notifier>)
  n189 = Unbundle By Name(w1) -> ("Notifiers.Async.ACQ HWAsync1"=w27:refnum<notifier>)
  n190 = Unbundle By Name(w1) -> ("Notifiers.Async.ACQ HWAsync1"=w26:refnum<notifier>)
  n191 = Unbundle By Name(w1) -> ("Notifiers.Async.ACQ HWAsync1"=w25:refnum<notifier>)
  n192 = while {
    tunnel: w138 -> [w570]
    tunnel: w131 -> [w564]
    tunnel: w101 -> [w549]
    tunnel: w100 -> [w548]
    tunnel: w99 -> [w547]
    tunnel: w98 -> [w546]
    tunnel: w57 -> [w483]
    tunnel: w97 -> [w515]
    tunnel: w96 -> [w514]
    tunnel: w95 -> [w513]
    tunnel: w94 -> [w512]
    tunnel: w93 -> [w511]
    tunnel: w24 -> [w485]
    stop <- w565 continue-if-true
    w484 = 200  # Timeout(ms)
    # "Display Loop"
    n193 = call "Wait on Async ACQ Notification.vi"("error in (no error)"=w483, "timeout in ms (-1)"=w484, "Async ACQ Notifier in"=w485) -> ("timed out?"=w478:bool, "Async ACQ"=w481:T10)  [unwired: 5 in, 2 out]
    n194 = call "Wait on ACQ Notification.vi"("error in (no error)"=w483, "timeout in ms (-1)"=w484, "ACQ Data Notifier in"=w570) -> ("timed out?"=w477:bool, "1 Sample"=w563:T11)  [unwired: 5 in, 2 out]
    n195 = call "Wait on ACQ Notification.vi"("error in (no error)"=w483, "timeout in ms (-1)"=w484, "ACQ Data Notifier in"=w549) -> ("timed out?"=w476:bool, "1 Sample"=w561:T11)  [unwired: 5 in, 2 out]
    n196 = call "Wait on ACQ Notification.vi"("error in (no error)"=w483, "timeout in ms (-1)"=w484, "ACQ Data Notifier in"=w548) -> ("timed out?"=w475:bool, "1 Sample"=w556:T11)  [unwired: 5 in, 2 out]
    n197 = call "Wait on ACQ Notification.vi"("error in (no error)"=w483, "timeout in ms (-1)"=w484, "ACQ Data Notifier in"=w547) -> ("timed out?"=w474:bool, "1 Sample"=w555:T11)  [unwired: 5 in, 2 out]
    n198 = call "Wait on ACQ Notification.vi"("error in (no error)"=w483, "timeout in ms (-1)"=w484, "ACQ Data Notifier in"=w546) -> ("timed out?"=w473:bool, "1 Sample"=w550:T11)  [unwired: 5 in, 2 out]
    n199 = call "Wait on CTRL Notification.vi"("error in (no error)"=w483, "timeout in ms (-1)"=w484, "CTRL Data Notifier in"=w515) -> ("timed out?"=w472:bool, "Control Data"=w562:T12)  [unwired: 5 in, 2 out]
    n200 = call "Wait on CTRL Notification.vi"("error in (no error)"=w483, "timeout in ms (-1)"=w484, "CTRL Data Notifier in"=w514) -> ("timed out?"=w471:bool, "Control Data"=w543:T12)  [unwired: 5 in, 2 out]
    n201 = call "Wait on CTRL Notification.vi"("error in (no error)"=w483, "timeout in ms (-1)"=w484, "CTRL Data Notifier in"=w513) -> ("timed out?"=w470:bool, "Control Data"=w538:T12)  [unwired: 5 in, 2 out]
    n202 = call "Wait on CTRL Notification.vi"("error in (no error)"=w483, "timeout in ms (-1)"=w484, "CTRL Data Notifier in"=w512) -> ("timed out?"=w469:bool, "Control Data"=w537:T12)  [unwired: 5 in, 2 out]
    n203 = call "Wait on CTRL Notification.vi"("error in (no error)"=w483, "timeout in ms (-1)"=w484, "CTRL Data Notifier in"=w511) -> ("timed out?"=w468:bool, "Control Data"=w532:T12)  [unwired: 5 in, 2 out]
    n204 = Wait on Occurrence(1:FALSE ("ignore previous (T)"), 2:w564, 3:w484) -> (0:w565:bool)
    n205 = feedback #2(w481) -> (w482:T10)
    n206 = Select(t=w482, s=w478, f=w481) -> (s? t:f=w480:T10)
    n207 = feedback-in #2(w480) -> ()
    n208 = feedback #3(w562) -> (w569:T12)
    n209 = Select(t=w569, s=w472, f=w562) -> (s? t:f=w568:T12)
    n210 = feedback-in #3(w568) -> ()
    n211 = feedback #4(w543) -> (w541:T12)
    n212 = Select(t=w541, s=w471, f=w543) -> (s? t:f=w542:T12)
    n213 = feedback-in #4(w542) -> ()
    n214 = feedback #5(w538) -> (w540:T12)
    n215 = Select(t=w540, s=w470, f=w538) -> (s? t:f=w539:T12)
    n216 = feedback-in #5(w539) -> ()
    n217 = feedback #6(w537) -> (w535:T12)
    n218 = Select(t=w535, s=w469, f=w537) -> (s? t:f=w536:T12)
    n219 = feedback-in #6(w536) -> ()
    n220 = feedback #7(w532) -> (w534:T12)
    n221 = Select(t=w534, s=w468, f=w532) -> (s? t:f=w533:T12)
    n222 = feedback-in #7(w533) -> ()
    n223 = feedback #8(w563) -> (w567:T11)
    n224 = Select(t=w567, s=w477, f=w563) -> (s? t:f=w566:T11)
    n225 = feedback-in #8(w566) -> ()
    n226 = feedback #9(w561) -> (w559:T11)
    n227 = Select(t=w559, s=w476, f=w561) -> (s? t:f=w560:T11)
    n228 = feedback-in #9(w560) -> ()
    n229 = feedback #10(w556) -> (w558:T11)
    n230 = Select(t=w558, s=w475, f=w556) -> (s? t:f=w557:T11)
    n231 = feedback-in #10(w557) -> ()
    n232 = feedback #11(w555) -> (w553:T11)
    n233 = Select(t=w553, s=w474, f=w555) -> (s? t:f=w554:T11)
    n234 = feedback-in #11(w554) -> ()
    n235 = feedback #12(w550) -> (w552:T11)
    n236 = Select(t=w552, s=w473, f=w550) -> (s? t:f=w551:T11)
    n237 = feedback-in #12(w551) -> ()
    n238 = Unbundle By Name(w480) -> ("Data"=→"Async Data":sgl[])
    n239 = Unbundle By Name(w566) -> ("TDX"=w493:sgl[])
    n240 = Unbundle By Name(w560) -> ("TDX"=w492:sgl[])
    n241 = Unbundle By Name(w557) -> ("TDX"=w491:sgl[])
    n242 = Unbundle By Name(w554) -> ("TDX"=w490:sgl[])
    n243 = Unbundle By Name(w551) -> ("TDX"=w489:sgl[])
    n244 = Unbundle By Name(w568) -> ("Encoder"=w545:sgl, "DI"=w527:bool[], "DO"=w519:bool[])
    n245 = Unbundle By Name(w542) -> ("Encoder"=w531:sgl, "DI"=w526:bool[], "DO"=w520:bool[])
    n246 = Unbundle By Name(w539) -> ("Encoder"=w530:sgl, "DI"=w525:bool[], "DO"=w521:bool[])
    n247 = Unbundle By Name(w536) -> ("Encoder"=w529:sgl, "DI"=w524:bool[], "DO"=w518:bool[])
    n248 = Unbundle By Name(w533) -> ("Encoder"=w528:sgl, "DI"=w523:bool[], "DO"=w517:bool[])
    n249 = Array Size(array=w493) -> (size(s)=w508:i32)
    n250 = Initialize Array(sgl 0.0 ("element"), w508) -> (w506:sgl[])
    n251 = Build Array(w545, w531, w530, w529, w528) -> (→"Encoder":sgl[])
    n252 = Build Array(w527, w526, w525, w524, w523) -> (→"DI":bool[][])
    n253 = Build Array(w519, w520, w521, w518, w517) -> (→"DO":bool[][])
    n254 = Build Array (concatenate)(w506, w492) -> (w502:sgl[])
    n255 = Array Size(array=w502) -> (size(s)=w503:i32)
    n256 = Initialize Array(sgl 0.0 ("element"), w503) -> (w505:sgl[])
    n257 = Build Array (concatenate)(w505, w491) -> (w499:sgl[])
    n258 = Array Size(array=w499) -> (size(s)=w498:i32)
    n259 = Initialize Array(sgl 0.0 ("element"), w498) -> (w500:sgl[])
    n260 = Build Array (concatenate)(w500, w490) -> (w488:sgl[])
    n261 = Array Size(array=w488) -> (size(s)=w497:i32)
    n262 = Initialize Array(sgl 0.0 ("element"), w497) -> (w496:sgl[])
    n263 = Build Array (concatenate)(w496, w489) -> (w494:sgl[])
    n264 = Build Array(w493, w492, w491, w490, w489) -> (w487:sgl[][])
    n265 = Number To Fractional String(number=w487) -> (F-format string=→"TDX ALL":string[][])  [unwired: 3 in]
    n266 = Build Array(w493, w502, w499, w488, w494) -> (→"TDX":sgl[][])
  }
  n267 = while {
    tunnel: w35 -> [w571]
    tunnel: w146 -> [w584]
    shift-right: [w576] -> _
    shift-left: w40 -> [w578]
    shift-right: [w574] -> _
    shift-left: w43 -> [w575]
    tunnel: w57 -> [w580]
    tunnel: [w581] -> w92
    shift-right: [w572] -> _
    shift-left: w43 -> [w573]
    stop <- w583 stop-if-true
    # "Logging Loop"
    n268 = call "Dequeue Message.vi"("error in (no error)"=w580, "Message Queue"=w584) -> ("error out"=w582:errorcluster, "Message Data"=w577:variant, "Message"=w585:string, "dup Message Queue"=w579:refnum<queue>)  [unwired: 6 in]
    n269 = case shown="\"Open Log File\"" w585 {
      tunnel: w579 -> [_ _ _ _ _ _]
      tunnel: [_ _ _ _ _ TRUE] -> w583
      tunnel: w582 -> [w589 w594 w605 w615 w621 w625]
      tunnel: [w589 w593 w604 w614 w621 w625] -> w581
      tunnel: w578 -> [w588 w591 w606 w616 w620 w624]
      tunnel: [w588 w590 w606 w616 w620 w624] -> w576
      tunnel: w577 -> [_ w592 w603 w613 _ _]
      tunnel: w575 -> [w586 w596 w600 w607 w619 w622]
      tunnel: [w586 w596 w598 w607 w619 w622] -> w574
      tunnel: w573 -> [w587 w595 w597 w609 w618 w623]
      tunnel: [w587 w595 w597 w608 w618 w623] -> w572
      tunnel: w571 -> [_ _ _ _ w617 _]
      frame Default {
      }
      frame "Update HAL Config" {
        n270 = Variant To Data(error in=w594, type=w591, Variant=w592) -> (data=w590:T1[], error out=w593:errorcluster)
      }
      frame "Start Time" {
        n271 = Variant To Data(error in=w605, type=u32 0, Variant=w603) -> (data=w601:u32, error out=w604:errorcluster)
        n272 = Get Date/Time In Seconds() -> (seconds since 1Jan1904=w599:timestamp)
        n273 = Replace Array Subset(array=w600, new element=w599, index=w601) -> (w598:timestamp[])
      }
      frame "Stop Time" {
        n274 = Variant To Data(error in=w615, type=u32 0, Variant=w613) -> (data=w611:u32, error out=w614:errorcluster)
        n275 = Get Date/Time In Seconds() -> (seconds since 1Jan1904=w610:timestamp)
        n276 = Replace Array Subset(array=w609, new element=w610, index=w611) -> (w608:timestamp[])
      }
      frame "Open Log File" {
        n277 = call "CreateLogFile.vi"("Stop Time"=w618, "Start Time"=w619, "HAL Config"=w620, "ACQ Queues"=w617) -> ()  [unwired: 8 in]
      }
      frame "EXIT" {
      }
    }
  }
  n278 = Unbundle By Name(w1) -> ("Notifiers.Acquisition.ACQ HWSync1"=w141:refnum<notifier>, "Notifiers.Control.CTRL HWSync1"=w140:refnum<notifier>, "Queues.ACQ HWSync1"=w139:refnum<queue>)
  n279 = Unbundle By Name(w1) -> ("Notifiers.Acquisition.ACQ HWSync2"=w128:refnum<notifier>, "Notifiers.Control.CTRL HWSync2"=w129:refnum<notifier>, "Queues.ACQ HWSync2"=w130:refnum<queue>)
  n280 = Unbundle By Name(w1) -> ("Notifiers.Acquisition.ACQ HWSync3"=w116:refnum<notifier>, "Notifiers.Control.CTRL HWSync3"=w117:refnum<notifier>, "Queues.ACQ HWSync3"=w118:refnum<queue>)
  n281 = Unbundle By Name(w1) -> ("Notifiers.Acquisition.ACQ HWSync4"=w121:refnum<notifier>, "Notifiers.Control.CTRL HWSync4"=w120:refnum<notifier>, "Queues.ACQ HWSync4"=w119:refnum<queue>)
  n282 = Unbundle By Name(w1) -> ("Notifiers.Acquisition.ACQ HWSync5"=w110:refnum<notifier>, "Notifiers.Control.CTRL HWSync5"=w111:refnum<notifier>, "Queues.ACQ HWSync5"=w112:refnum<queue>)
  n283 = call "AutoMeasurement.vi"("index"=4 ("line index"), "CTRL HWSync"=w9, "HAL"=w8, "Queue in"=w7) -> ()  [unwired: 8 in]
  n284 = call "AutoMeasurement.vi"("index"=5 ("line index"), "CTRL HWSync"=w4, "HAL"=w5, "Queue in"=w6) -> ()  [unwired: 8 in]
  n285 = call "AutoMeasurement.vi"("index"=1 ("line index"), "CTRL HWSync"=w20, "HAL"=w21, "Queue in"=w22) -> ()  [unwired: 8 in]
  n286 = call "AutoMeasurement.vi"("index"=3 ("line index"), "CTRL HWSync"=w12, "HAL"=w13, "Queue in"=w14) -> ()  [unwired: 8 in]
  n287 = call "AutoMeasurement.vi"("index"=2 ("line index"), "CTRL HWSync"=w17, "HAL"=w16, "Queue in"=w15) -> ()  [unwired: 8 in]
  n288 = Unbundle By Name(w2) -> ("HAL"=w70:refnum<queue>, "HWAsync10"=w71:refnum<queue>)
  n289 = Unbundle By Name(w2) -> ("HAL"=w87:refnum<queue>, "HWAsync1"=w86:refnum<queue>)
  n290 = Unbundle By Name(w2) -> ("HAL"=w82:refnum<queue>, "HWAsync2"=w83:refnum<queue>)
  n291 = Unbundle By Name(w2) -> ("HAL"=w81:refnum<queue>, "HWAsync3"=w80:refnum<queue>)
  n292 = Unbundle By Name(w2) -> ("HAL"=w76:refnum<queue>, "HWAsync4"=w77:refnum<queue>)
  n293 = Unbundle By Name(w2) -> ("HAL"=w75:refnum<queue>, "HWAsync5"=w74:refnum<queue>)
  n294 = Unbundle By Name(w2) -> ("HAL"=w58:refnum<queue>, "HWAsync6"=w59:refnum<queue>)
  n295 = Unbundle By Name(w2) -> ("HAL"=w63:refnum<queue>, "HWAsync7"=w62:refnum<queue>)
  n296 = Unbundle By Name(w2) -> ("HAL"=w64:refnum<queue>, "HWAsync8"=w65:refnum<queue>)
  n297 = Unbundle By Name(w2) -> ("HAL"=w69:refnum<queue>, "HWAsync9"=w68:refnum<queue>)
  n298 = Unbundle By Name(w2) -> ("HAL"=w151:refnum<queue>, "HWSync1"=w150:refnum<queue>)
  n299 = Unbundle By Name(w2) -> ("HAL"=w125:refnum<queue>, "HWSync2"=w126:refnum<queue>)
  n300 = Unbundle By Name(w2) -> ("HAL"=w113:refnum<queue>, "HWSync3"=w114:refnum<queue>)
  n301 = Unbundle By Name(w2) -> ("HAL"=w124:refnum<queue>, "HWSync4"=w123:refnum<queue>)
  n302 = Unbundle By Name(w2) -> ("HAL"=w107:refnum<queue>, "HWSync5"=w108:refnum<queue>)
  n303 = call "HWSyncLoop.vi"("HAL"=w151, "Index"=u32 1 ("Num of Loop"), "HWSync"=w150, "error in"=w57, "ACQ Data Queue"=w139, "CTRL Data Notifier"=w140, "ACQ Data Notifier"=w141) -> ("error out"=w106:errorcluster)  [unwired: 4 in]
  n304 = call "HWSyncLoop.vi"("HAL"=w125, "Index"=u32 2 ("Num of Loop"), "HWSync"=w126, "error in"=w57, "ACQ Data Queue"=w130, "CTRL Data Notifier"=w129, "ACQ Data Notifier"=w128) -> ("error out"=w105:errorcluster)  [unwired: 4 in]
  n305 = call "HWSyncLoop.vi"("HAL"=w113, "Index"=u32 3 ("Num of Loop"), "HWSync"=w114, "error in"=w57, "ACQ Data Queue"=w118, "CTRL Data Notifier"=w117, "ACQ Data Notifier"=w116) -> ("error out"=w104:errorcluster)  [unwired: 4 in]
  n306 = call "HWSyncLoop.vi"("HAL"=w124, "Index"=u32 4 ("Num of Loop"), "HWSync"=w123, "error in"=w57, "ACQ Data Queue"=w119, "CTRL Data Notifier"=w120, "ACQ Data Notifier"=w121) -> ("error out"=w103:errorcluster)  [unwired: 4 in]
  n307 = call "HWSyncLoop.vi"("HAL"=w107, "Index"=u32 5 ("Num of Loop"), "HWSync"=w108, "error in"=w57, "ACQ Data Queue"=w112, "CTRL Data Notifier"=w111, "ACQ Data Notifier"=w110) -> ("error out"=w102:errorcluster)  [unwired: 4 in]
  n308 = call "HWAsyncLoop.vi"("HAL"=w87, "Index"=u32 1, "HWAsync"=w86, "error in"=w57, "Async ACQ Notifier in"=w34) -> ("error out"=w56:errorcluster)  [unwired: 6 in]
  n309 = call "HWAsyncLoop.vi"("HAL"=w82, "Index"=u32 2, "HWAsync"=w83, "error in"=w57, "Async ACQ Notifier in"=w33) -> ("error out"=w54:errorcluster)  [unwired: 6 in]
  n310 = call "HWAsyncLoop.vi"("HAL"=w81, "Index"=u32 3, "HWAsync"=w80, "error in"=w57, "Async ACQ Notifier in"=w32) -> ("error out"=w53:errorcluster)  [unwired: 6 in]
  n311 = call "HWAsyncLoop.vi"("HAL"=w76, "Index"=u32 4, "HWAsync"=w77, "error in"=w57, "Async ACQ Notifier in"=w31) -> ("error out"=w52:errorcluster)  [unwired: 6 in]
  n312 = call "HWAsyncLoop.vi"("HAL"=w75, "Index"=u32 5, "HWAsync"=w74, "error in"=w57, "Async ACQ Notifier in"=w30) -> ("error out"=w51:errorcluster)  [unwired: 6 in]
  n313 = call "HWAsyncLoop.vi"("HAL"=w58, "Index"=u32 6, "HWAsync"=w59, "error in"=w57, "Async ACQ Notifier in"=w29) -> ("error out"=w50:errorcluster)  [unwired: 6 in]
  n314 = call "HWAsyncLoop.vi"("HAL"=w63, "Index"=u32 7, "HWAsync"=w62, "error in"=w57, "Async ACQ Notifier in"=w28) -> ("error out"=w49:errorcluster)  [unwired: 6 in]
  n315 = call "HWAsyncLoop.vi"("HAL"=w64, "Index"=u32 8, "HWAsync"=w65, "error in"=w57, "Async ACQ Notifier in"=w27) -> ("error out"=w48:errorcluster)  [unwired: 6 in]
  n316 = call "HWAsyncLoop.vi"("HAL"=w69, "Index"=u32 9, "HWAsync"=w68, "error in"=w57, "Async ACQ Notifier in"=w26) -> ("error out"=w47:errorcluster)  [unwired: 6 in]
  n317 = call "HWAsyncLoop.vi"("HAL"=w70, "Index"=u32 10, "HWAsync"=w71, "error in"=w57, "Async ACQ Notifier in"=w25) -> ("error out"=w46:errorcluster)  [unwired: 6 in]
  n318 = Merge Errors(w56, w54, w53, w52, w51, w50, w49, w48, w47, w46) -> (w55:errorcluster)
  n319 = Set Occurrence(w132) -> ()
  n320 = Merge Errors(w106, w105, w104, w103, w102, w55) -> (w91:errorcluster)
  n321 = Merge Errors(w149, w90, w91, w92) -> (w137:errorcluster)
  n322 = call "Destroy All Data Queues.vi"("Error In"=w137, "WINFAS 2 Data Queue.lvlib:All Data Queues Cluster"=w1) -> ("Error Out"=w136:errorcluster)  [unwired: 9 in]
  n323 = call "Destroy All Message Queues.vi"("error in (no error)"=w136, "Message Queues Out"=w2) -> ("error out"=w135:errorcluster)  [unwired: 9 in]
  n324 = property class="App"(error in=w135) -> ("App.Kind"=w145:T2)  [unwired: 1 in, 2 out]
  n325 = case shown="\"Development System\"" w145 {
    tunnel: [TRUE FALSE TRUE] -> w144
    tunnel: [w627 w641 w647] -> _
    frame "invalid app kind", Default {
      n326 = property class="VI"() -> (error out=w628:errorcluster, "Panel"=w638:refnum<vi>)  [unwired: 2 in, 1 out]
      n327 = property class="Pnl"(reference=w638, error in=w628) -> (error out=w629:errorcluster, "AllObjs[]"=w637:refnum<vi>[])  [unwired: 1 out]
      n328 = control-ref of="This VI"() -> (w635:refnum<vi>)
      n329 = Close Reference(reference=w637, error in (no error)=w629) -> (error out=w634:errorcluster)
      n330 = invoke class="VI" method="FP.Close"(reference=w635, error in=w634) -> (reference out=w633:refnum<vi>, error out=w632:errorcluster)  [unwired: 1 in, 1 out]
      n331 = invoke class="VI" method="Abort VI"(reference=w633, error in=w632) -> (reference out=w630:refnum<vi>, error out=w631:errorcluster)  [unwired: 1 in, 1 out]
      n332 = Close Reference(reference=w630, error in (no error)=w631) -> (error out=w639:errorcluster)
      n333 = control-ref of="This Application"() -> (w640:refnum<vi>)
      n334 = Close Reference(reference=w640, error in (no error)=w639) -> (error out=w627:errorcluster)
    }
    frame "Development System" {
      n335 = property class="VI"() -> (error out=w642:errorcluster, "Panel"=w646:refnum<vi>)  [unwired: 2 in, 1 out]
      n336 = property class="Pnl"(reference=w646, error in=w642) -> (error out=w643:errorcluster, "AllObjs[]"=w645:refnum<vi>[])  [unwired: 1 out]
      n337 = Close Reference(reference=w645, error in (no error)=w643) -> (error out=w641:errorcluster)
    }
    frame "Run Time System" {
      n338 = property class="VI"() -> (error out=w648:errorcluster, "Panel"=w658:refnum<vi>)  [unwired: 2 in, 1 out]
      n339 = property class="Pnl"(reference=w658, error in=w648) -> (error out=w649:errorcluster, "AllObjs[]"=w657:refnum<vi>[])  [unwired: 1 out]
      n340 = control-ref of="This VI"() -> (w655:refnum<vi>)
      n341 = Close Reference(reference=w657, error in (no error)=w649) -> (error out=w654:errorcluster)
      n342 = invoke class="VI" method="FP.Close"(reference=w655, error in=w654) -> (reference out=w653:refnum<vi>, error out=w652:errorcluster)  [unwired: 1 in, 1 out]
      n343 = invoke class="VI" method="Abort VI"(reference=w653, error in=w652) -> (reference out=w650:refnum<vi>, error out=w651:errorcluster)  [unwired: 1 in, 1 out]
      n344 = Close Reference(reference=w650, error in (no error)=w651) -> (error out=w659:errorcluster)
      n345 = control-ref of="This Application"() -> (w660:refnum<vi>)
      n346 = Close Reference(reference=w660, error in (no error)=w659) -> (error out=w647:errorcluster)
    }
  }
  n347 = Quit LabVIEW(quit? (T)=w144) -> ()
